vi "Get Bucket Location.vi"(8 "error in (no error)":errorcluster, 11 "Bucket in":refnum<class "Bucket.lvclass">) -> (0 "error out":errorcluster, 2 "Location":T1, 3 "Bucket out":refnum<class "Bucket.lvclass">)   [LabVIEW 2015, in "NI_AWS_S3.lvlib" / "Bucket.lvclass"]
doc: "This implementation of the GET operation uses the location subresource to return a bucket's region. You set the bucket's region using the LocationConstraint request parameter in a PUT Bucket request. To use this implementation of the operation, you must be the bucket owner."
uses:
  Bucket.lvclass
  Core/HTTP Request/Region.ctl
  Core/HTTP Request/Request Options.ctl
  Core/HTTP Request/Name Value Pair.ctl
  Core/HTTP Request/Region handling.ctl
  Core/HTTP Request/URL formatting.ctl
  Bucket.lvclass/Bucket.ctl
  Read Name.vi
  Core/HTTP Request/HTTP Request.lvclass
  XML Parsing/NI_XML Parsing.lvlib
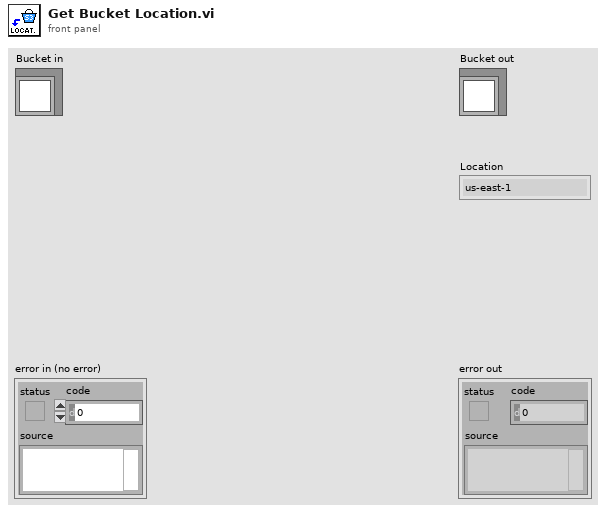
[diagram p1: front panel]
types:
  T1 = typedef "NI_AWS_Core.lvlib/HTTP Request.lvclass/Region.ctl" = enum16{"us-east-1", "us-east-2", "us-west-1", "us-west-2", "ap-northeast-1", "ap-northeast-2", "ap-southeast-1", "ap-southeast-2", "ca-central-1", "eu-central-1", "eu-west-1", "eu-west-2", "sa-east-1"}
  T2 = typedef "NI_AWS_Core.lvlib/HTTP Request.lvclass/URL formatting.ctl" = enum16{"region-", "region."}
  T3 = typedef "NI_AWS_Core.lvlib/HTTP Request.lvclass/Region handling.ctl" = enum16{"use region everywhere", "use region (authentication only)", "use region (URL only)", "ignore region everwhere"}
  T4 = typedef "NI_AWS_Core.lvlib/HTTP Request.lvclass/Name Value Pair.ctl" = cluster{"name":string, "value":string}
  T5 = typedef "NI_AWS_Core.lvlib/HTTP Request.lvclass/Request Options.ctl" = cluster{"request headers":T4[], "request parameters":T4[], "request body":string, "region handling":T3, "URL formatting":T2}
  T6 = typedef "NI_AWS_Core.lvlib/HTTP Request.lvclass/Response.ctl" = cluster{"Headers":string, "Body":string}
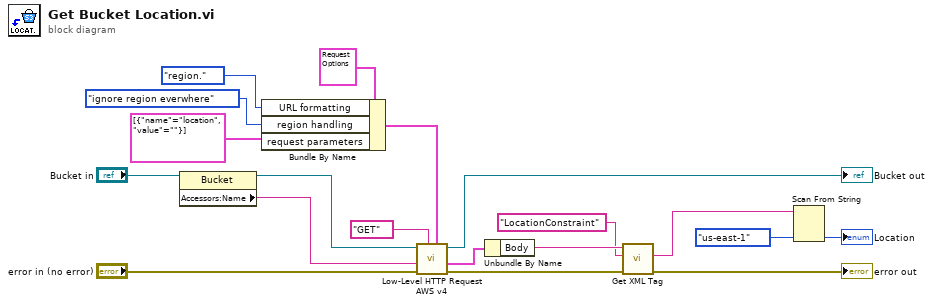
[diagram p0: block diagram]
diagram:
  n1 = property class="Bucket"(reference="Bucket in") -> (reference out=w5:refnum<class "Bucket.lvclass">, "Accessors:Name"=w1:string)  [unwired: 1 in, 1 out]
  n2 = Bundle By Name(cluster=T5 {"request headers"=[], "request parameters"=[], "request body"="", "region handling"=enum."use region everywhere", "URL formatting"=enum."region."} ("Request Options"), "URL formatting"=URL_formatting."region.", "region handling"=Region_handling."ignore region everwhere", "request parameters"=T4[] [{"name"="location", "value"=""}]) -> (w2:T5)
  n3 = call "Low-Level HTTP Request AWS v4.vi"("Request Options"=w2, "HTTP-Verb"="GET", "error in (no error)"="error in (no error)", "URL Suffix"=w1, "AWS Core in"=w5) -> ("error out"=w15:errorcluster, "Response"=w3:T6, "AWS Core out"=→"Bucket out":refnum<class "Bucket.lvclass">)  [unwired: 3 in, 1 out]
  n4 = Unbundle By Name(w3) -> ("Body"=w16:string)
  n5 = call "Get XML Tag.vi"("error in (no error)"=w15, "Tag name"="LocationConstraint", "XML String in"=w16) -> ("error out"=→"error out":errorcluster, "Tag value"=w12:string)  [unwired: 4 in, 3 out]
  n6 = Scan From String(input string=w12, default 1=Region."us-east-1" ("Region")) -> (output 1=→"Location":T1)  [unwired: 3 in, 3 out]
